vi "Дешифратор клавиатуры.vi"(3 "-":bool, 4 "R":bool, 5 "C":bool, 6 "Input":T3) -> (0 "-":bool, 1 "Един":T1, 2 "Дес":T2)   [LabVIEW 2017]
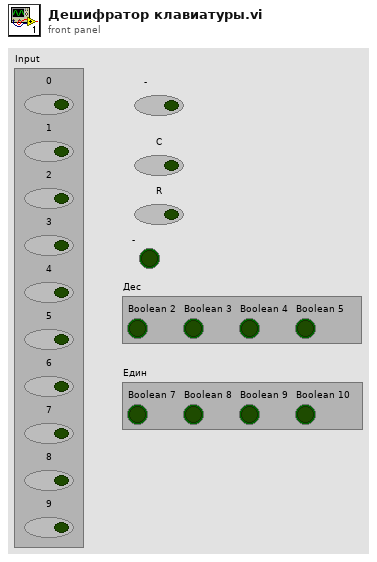
[diagram p1: front panel]
types:
  T1 = cluster{"Boolean 7":bool, "Boolean 8":bool, "Boolean 9":bool, "Boolean 10":bool}
  T2 = cluster{"Boolean 2":bool, "Boolean 3":bool, "Boolean 4":bool, "Boolean 5":bool}
  T3 = cluster{"0":bool, "1":bool, "2":bool, "3":bool, "4":bool, "5":bool, "6":bool, "7":bool, "8":bool, "9":bool}
  T4 = cluster{"Q3":bool, "Q2":bool, "Q1":bool, "Q0":bool}
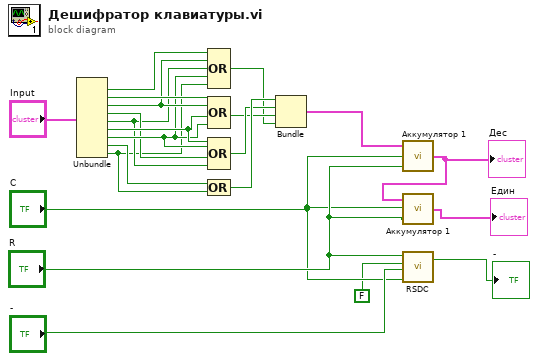
[diagram p0: block diagram]
diagram:
  n1 = Unbundle("Input") -> ("1"=w21:bool, "2"=w20:bool, "3"=w19:bool, "4"=w16:bool, "5"=w15:bool, "6"=w18:bool, "7"=w17:bool, "8"=w14:bool, "9"=w13:bool)  [unwired: 1 out]
  n2 = Compound Arithmetic op=OR(w21, w19, w15, w17, w13) -> (w9:bool)
  n3 = Compound Arithmetic op=OR(w20, w19, w18, w17) -> (w10:bool)
  n4 = Compound Arithmetic op=OR(w18, w17, w16, w15) -> (w11:bool)
  n5 = Compound Arithmetic op=OR(w14, w13) -> (w12:bool)
  n6 = Bundle(w12, w11, w10, w9) -> (w8:cluster{bool, bool, bool, bool})  [unwired: 1 in]
  n7 = call "Аккумулятор 1.vi"("Reset"="R", "C"="C", "d"=w8) -> ("output"=w6:T4)
  "Дес" <- w6
  n8 = call "Аккумулятор 1.vi"("Reset"="R", "C"="C", "d"=w6) -> ("output"=→"Един":T4)
  n9 = call "RSDC.vi"("c"="C", "d"="-", "s"=FALSE, "r"="R") -> ("q"=→"-":bool)  [unwired: 1 out]
